vi "Trata PDA.vi"() -> ()   [LabVIEW 2018]
uses:
  tele.llb/TCSPD Globals.vi
  Global_Telescopio.vi
panel:
  in  "Case Constant\n(See Context Help)":bool=TRUE
  out "DEC PDA":dbl format="%#.9f"
  out "AH PDA":dbl format="%#.9f"
  out "CoordDEC":bool
  out "CoordAH":bool
  out "String":string
  out "Equipamento":string
  out "Comando":string
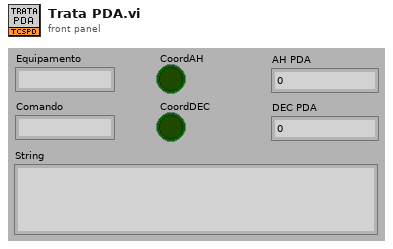
[diagram p1: front panel]
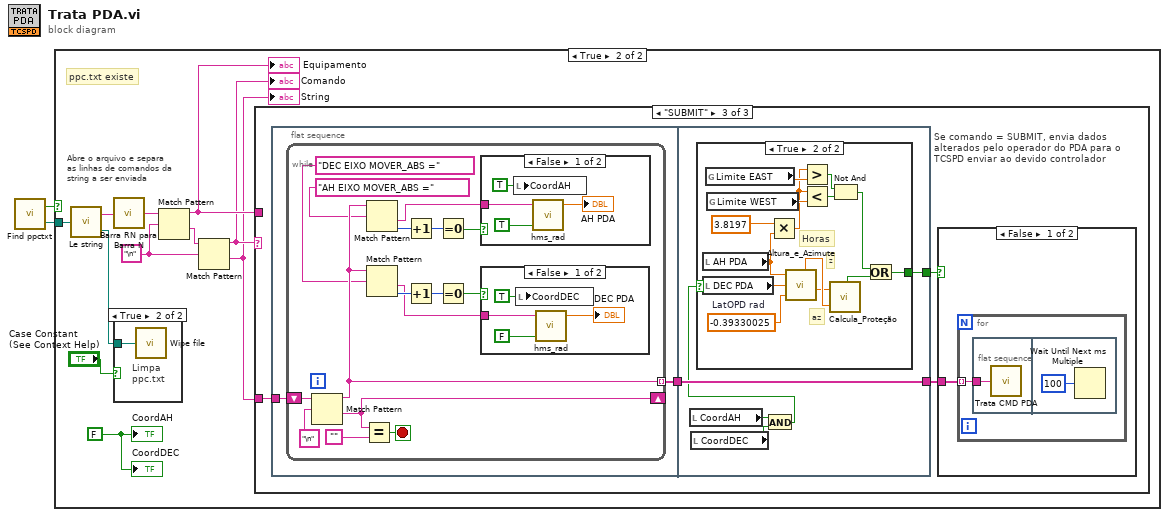
[diagram p0: block diagram]
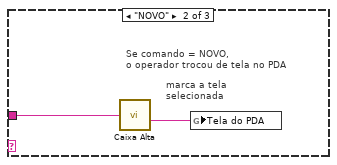
[diagram p5: hidden frame]
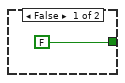
[diagram p8: hidden frame]
diagram:
  n1 = call "Find ppctxt.vi"() -> ("Existe ppc.txt?"=w1:bool, "ppc.txt Path"=w2:path)  [unwired: 1 in]
  n2 = case shown="True" w1 {
    tunnel: w2 -> [_ w13]
    frame False {
      # "ppc.txt não existe"
    }
    frame True {
      w4 = FALSE
      w3 = "\n" ("regular expression")
      # "ppc.txt existe"
      # "Abre o arquivo e separa\nas linhas de comandos da\nstring a ser enviada"
      n3 = call "Le string.vi"("path in"=w13) -> ("saida"=w12:string, "path out"=w9:path)
      n4 = call "Barra RN para Barra N.vi"("Input string"=w12) -> ("Output string"=w5:string)
      n5 = case shown="True" "Case Constant\n(See Context Help)" {
        tunnel: w9 -> [_ w14]
        frame False {
        }
        frame True {
          # "Limpa\nppc.txt"
          n6 = call "Wipe file.vi"("ppc path"=w14) -> ()  [unwired: 2 out]
        }
      }
      n7 = Match Pattern(string=w5, regular expression=w3) -> (before substring=w11:string, after substring=w8:string)  [unwired: 1 in, 2 out]
      "Equipamento" <- w11
      n8 = Match Pattern(string=w8, regular expression=w3) -> (before substring=w7:string, after substring=w6:string)  [unwired: 1 in, 2 out]
      "Comando" <- w7
      "String" <- w6
      n9 = case shown="\"SUBMIT\"" w7 {
        tunnel: w11 -> [_ w15 _]
        tunnel: w6 -> [_ _ w20]
        frame "", Default {
        }
        frame "NOVO" {
          # "Se comando = NOVO,\no operador trocou de tela no PDA"
          # "marca a tela\nselecionada"
          n10 = call "Caixa Alta.vi"("String in"=w15) -> ("String out"=w16:string)
          n11 = global write "TCSPD Globals.vi" "Tela do PDA"(w16) -> ()
        }
        frame "SUBMIT" {
          # "Se comando = SUBMIT, envia dados alterados pelo operador do PDA para o TCSPD enviar ao devido controlador"
          n12 = flat-sequence {
            tunnel: w20 -> [w22]
            tunnel: [w21] -> w19
            tunnel: [w49] -> w18
            tunnel: w19 -> [w49]
            tunnel: [w48] -> w17
            frame #0 {
              n13 = while {
                shift-right: [w35] -> _
                shift-left: w22 -> [w37]
                tunnel: [w33] -> w21 mode=indexing
                stop <- w36 stop-if-true
                n14 = Match Pattern(string=w37, regular expression="\n") -> (before substring=w33:string, after substring=w35:string)  [unwired: 1 in, 2 out]
                n15 = Equal?(x=w35, y="") -> (x = y?=w36:bool)
                n16 = Match Pattern(string=w33, regular expression="AH EIXO MOVER_ABS =") -> (after substring=w24:string, offset past match=w29:i32)  [unwired: 1 in, 2 out]
                n17 = Match Pattern(string=w33, regular expression="DEC EIXO MOVER_ABS =") -> (after substring=w23:string, offset past match=w30:i32)  [unwired: 1 in, 2 out]
                n18 = Increment(x=w29) -> (x+1=w27:i32)
                n19 = Increment(x=w30) -> (x+1=w28:i32)
                n20 = Equal To 0?(x=w27) -> (x = 0?=w26:bool)
                n21 = Equal To 0?(x=w28) -> (x = 0?=w25:bool)
                n22 = case shown="False" w26 {
                  tunnel: w24 -> [w46 _]
                  frame False {
                    n23 = local write "CoordAH"(TRUE ("True = hora")) -> ()
                    n24 = call "hms_rad.vi"("True = hora"=TRUE, "Texto Graus"=w46) -> ("radianos"=→"AH PDA":dbl)  [unwired: 3 in]
                  }
                  frame True {
                  }
                }
                n25 = case shown="False" w25 {
                  tunnel: w23 -> [w42 _]
                  frame False {
                    n26 = local write "CoordDEC"(TRUE ("True = hora")) -> ()
                    n27 = call "hms_rad.vi"("True = hora"=FALSE, "Texto Graus"=w42) -> ("radianos"=→"DEC PDA":dbl)  [unwired: 3 in]
                  }
                  frame True {
                  }
                }
              }
            }
            frame #1 {
              n28 = local read "CoordAH"() -> (w51:bool)
              n29 = local read "CoordDEC"() -> (w50:bool)
              n30 = And(x=w51, y=w50) -> (x .and. y?=w47:bool)
              n31 = case shown="True" w47 {
                tunnel: [FALSE w55] -> w48
                frame False {
                }
                frame True {
                  w66 = -0.39330025  # LatOPD rad
                  # "Horas"
                  # "az"
                  # "z"
                  n32 = local read "AH PDA"() -> (w58:dbl)
                  n33 = local read "DEC PDA"() -> (w63:dbl)
                  n34 = global read "Global_Telescopio.vi" "Limite EAST"() -> (w61:dbl)
                  n35 = global read "Global_Telescopio.vi" "Limite WEST"() -> (w60:dbl)
                  n36 = Multiply(x=3.8197 ("y"), y=w58) -> (x*y=w59:dbl)
                  n37 = call "Altura_e_Azimute.vi"("LAT rad"=w66, "DEC rad"=w63, "AH rad"=w58) -> ("AZIMUTE rad"=w64:dbl, "ANG. ZENITAL rad"=w65:dbl)  [unwired: 4 out]
                  n38 = Greater?(x=w59, y=w61) -> (0:w56:bool)
                  n39 = Less?(x=w59, y=w60) -> (x < y?=w57:bool)
                  n40 = call "Calcula_Proteção.vi"("Zenital angle rad"=w65, "Azimute rad"=w64) -> ("Prot Zmax"=w53:bool)  [unwired: 4 out]
                  n41 = Not And(1:w57, 2:w56) -> (0:w54:bool)
                  n42 = Or(x=w54, y=w53) -> (x .or. y?=w55:bool)
                }
              }
            }
          }
          n43 = case shown="False" w17 {
            tunnel: w18 -> [w67 _]
            frame False {
              n44 = for {
                tunnel: w67 -> [w68] mode=indexing
                n45 = flat-sequence {
                  tunnel: w68 -> [w69]
                  frame #0 {
                    n46 = call "Trata CMD PDA.vi"("Comando"=w69) -> ()  [unwired: 4 in, 1 out]
                  }
                  frame #1 {
                    n47 = Wait Until Next ms Multiple(millisecond multiple=u32 100) -> ()  [unwired: 1 out]
                  }
                }
              }
            }
            frame True {
            }
          }
        }
      }
      "CoordAH" <- w4
      "CoordDEC" <- w4
    }
  }
